vi "HSV to RGB.vi"(3 "V":dbl, 4 "S":dbl, 5 "H":dbl) -> (0 "B":u8, 1 "G":u8, 2 "R":u8)   [LabVIEW 2014]
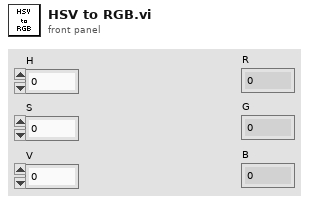
[diagram p1: front panel]
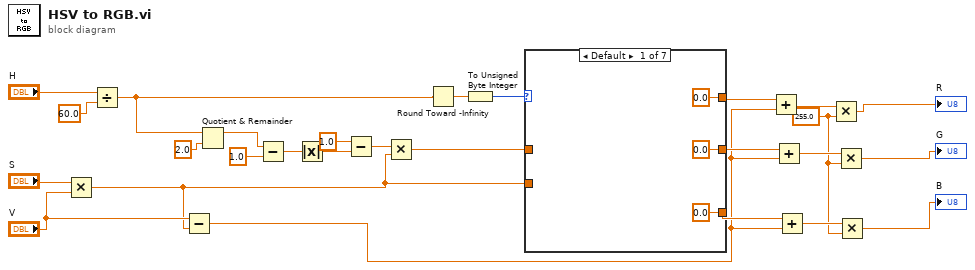
[diagram p0: block diagram]
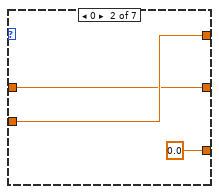
[diagram p2: hidden frame]
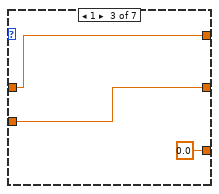
[diagram p3: hidden frame]
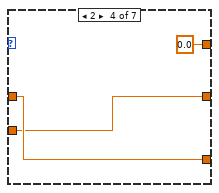
[diagram p4: hidden frame]
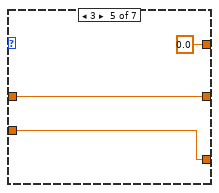
[diagram p5: hidden frame]
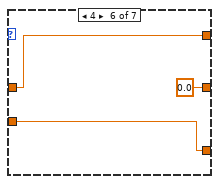
[diagram p6: hidden frame]
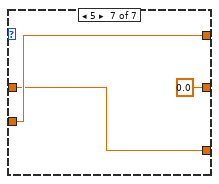
[diagram p7: hidden frame]
diagram:
  w5 = 255.0 ("y")
  n1 = Multiply(x="S", y="V") -> (x*y=w13:dbl)
  n2 = Divide(x="H", y=60.0) -> (x/y=w1:dbl)
  n3 = Subtract(x="V", y=w13) -> (x-y=w9:dbl)
  n4 = Quotient & Remainder(x=w1, y=2.0) -> (x-y*floor(x/y)=w24:dbl)  [unwired: 1 out]
  n5 = Subtract(x=w24, y=1.0) -> (x-y=w22:dbl)
  n6 = Absolute Value(x=w22) -> (abs(x)=w20:dbl)
  n7 = Subtract(x=1.0, y=w20) -> (x-y=w18:dbl)
  n8 = Multiply(x=w18, y=w13) -> (x*y=w15:dbl)
  n9 = Round Toward -Infinity(1:w1) -> (0:w17:dbl)
  n10 = To Unsigned Byte Integer(number=w17) -> (unsigned 8bit integer=w16:u8)
  n11 = case shown="Default" w16 {
    tunnel: w15 -> [_ w32 w36 w38 w41 w45 w46]
    tunnel: w13 -> [_ w33 w35 w37 w40 w43 w48]
    tunnel: [0.0 w33 w36 0.0 0.0 w45 w48] -> w12
    tunnel: [0.0 w32 w35 w37 w41 0.0 0.0] -> w11
    tunnel: [0.0 0.0 0.0 w38 w40 w43 w46] -> w10
    frame Default {
    }
    frame 0 {
    }
    frame 1 {
    }
    frame 2 {
    }
    frame 3 {
    }
    frame 4 {
    }
    frame 5 {
    }
  }
  n12 = Add(x=w12, y=w9) -> (x+y=w8:dbl)
  n13 = Add(x=w11, y=w9) -> (x+y=w7:dbl)
  n14 = Add(x=w10, y=w9) -> (x+y=w6:dbl)
  n15 = Multiply(x=w8, y=w5) -> (x*y=→"R":dbl)
  n16 = Multiply(x=w7, y=w5) -> (x*y=→"G":dbl)
  n17 = Multiply(x=w6, y=w5) -> (x*y=→"B":dbl)
